vi "ReadSignalFromTXT.vi"(8 "error in":errorcluster, 11 "file path in":path) -> (0 "error out":errorcluster, 3 "signal out":waveform(dbl)(graph))   [LabVIEW 2025]
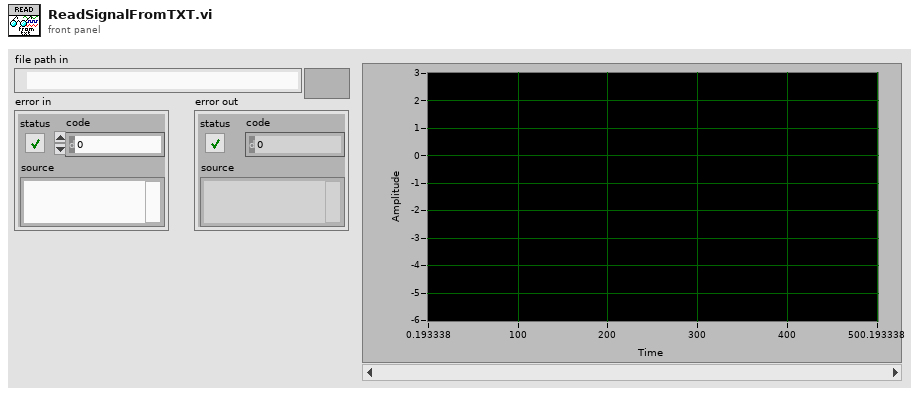
[diagram p1: front panel]
types:
  T1 = enum16{"open", "replace", "create", "open or create", "replace or create", "replace or create with confirmation"}
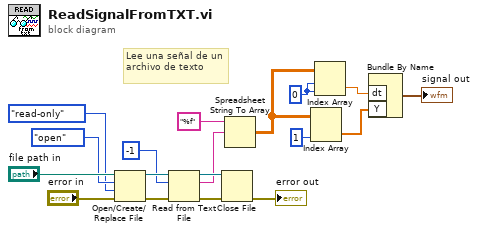
[diagram p0: block diagram]
diagram:
  w6 = 0
  # "Lee una señal de un archivo de texto"
  n1 = Open/Create/Replace File(file path (use dialog)="file path in", error in="error in", operation (0:open)=T1."open", access (0:read/write)=enum16{"read/write", "read-only", "write-only"}."read-only") -> (refnum out=w15:refnum<file>, error out=w13:errorcluster)  [unwired: 2 in, 1 out]
  n2 = Read from Text File(file (use dialog)=w15, count=-1, error in=w13) -> (refnum out=w12:refnum<file>, text=w8:string, error out=w11:errorcluster)  [unwired: 1 in, 1 out]
  n3 = Close File(refnum=w12, error in=w11) -> (error out=→"error out":errorcluster)  [unwired: 1 out]
  n4 = Spreadsheet String To Array(format string="%f", spreadsheet string=w8) -> (array=w3:dbl[][])  [unwired: 2 in]
  n5 = Index Array(array=w3, index (col)=1 ("index (row)")) -> (element=w1:dbl[])  [unwired: 1 in]
  n6 = Index Array(array=w3, index (row)=w6, index (col)=w6) -> (element=w5:dbl)
  n7 = Bundle By Name("dt"=w5, "Y"=w1) -> (→"signal out":waveform(dbl))  [unwired: 1 in]
